vi "Interface Benchmark.vi"() -> (3 "one-way latency":u64 format="%d us")   [LabVIEW 2017]
uses:
  <vilib>/Platform/TimedLoop/XDataNode/timing_clust.ctl
  <vilib>/Platform/TimedLoop/XDataNode/nitl_modes.ctl
  <vilib>/Platform/TimedLoop/XDataNode/wakeup.ctl
  <vilib>/platform/TimedLoop/XDataNode/XDataNode.xnode
  Classes/Interfaces/Dispatcher/Dispatcher Interface.lvclass
  <vilib>/Platform/TimedLoop/XDataNode/XDNodeRunTimeDep.lvlib
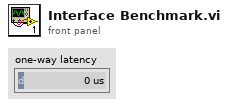
[diagram p1: front panel]
types:
  T1 = typedef "XDNodeRunTimeDep.lvlib/timing_clust.ctl" = cluster{"Expected End [f-1]":u64, "Actual End [f-1]":u64, "Finished Late? [f-1]":bool, "Expected End [i-1]":u64, "Actual End [i-1]":u64, "Finished Late? [i-1]":bool, "Expected Start [i]":u64, "Actual Start [i]":u64, "Expected Start [f]":u64, "Actual Start [f]":u64, "Source Name":string, "Structure Name":string, "Period":i64, "Deadline":i64, "Offset":i64, "Start":i64, "Priority":i32, "Timeout":i32, "Mode":T2, "Wakeup Reason":T3, "Error":errorcluster, "Source Type":string, "Secondary Source Type":string, "Global End Time":u64, "Global Start Time":u64, "Frame Duration":u64, "Iteration Duration":u64, "Assigned CPU":i32, "I/O Scan Engine Mode":u32}
  T2 = typedef "XDNodeRunTimeDep.lvlib/nitl_modes.ctl" = enum32{"No Change", "Process missed periods, maintain original phase", "Discard missed periods, maintain original phase", "Process missed periods, ignore original phase", "Discard missed periods, ignore original phase"}
  T3 = typedef "XDNodeRunTimeDep.lvlib/wakeup.ctl" = enum32{"Normal", "Aborted", "Asynchronous wakeup", "Timing source error", "Timed loop error", "Timeout"}
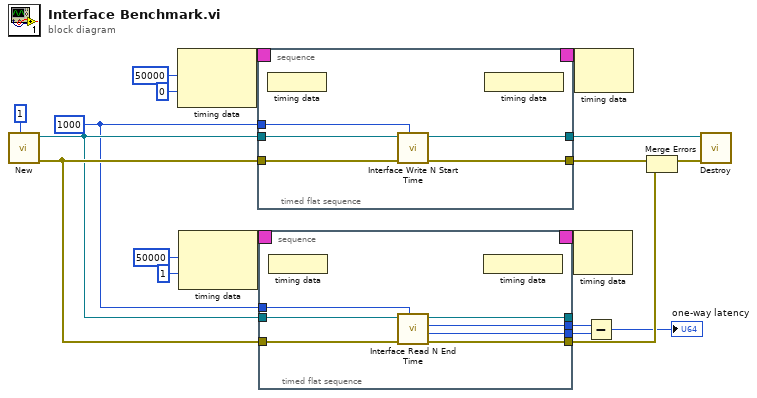
[diagram p0: block diagram]
diagram:
  w1 = 1000 ("count (1)")
  n1 = call "New.vi"("fifo depths (10)"=u32 1) -> ("error out"=w9:errorcluster, "Dispatcher Interface"=w8:refnum<class "Dispatcher Interface.lvclass">)  [unwired: 9 in]
  n2 = node-c288(50000 ("Priority"), 0 ("Processor")) -> (w15:T1)
  n3 = node-c288(50000 ("Priority"), 1 ("Processor")) -> (w12:T1)
  n4 = timed-sequence {
    timing: w15 -> [_]
    timing-out: [_] -> w14
    tunnel: [w24] -> w18
    tunnel: w9 -> [w23]
    tunnel: [w22] -> w17
    tunnel: w8 -> [w21]
    tunnel: w1 -> [w20]
    n5 = timed-flat-sequence {
      tunnel: [w29] -> w24
      tunnel: w23 -> [w28]
      tunnel: [w27] -> w22
      tunnel: w21 -> [w26]
      tunnel: w20 -> [w25]
      n6 = node-c288() -> ()  [unwired: 1 in]
      n7 = call "Interface Write N Start Time.vi"("count (1)"=w25, "error in (no error)"=w28, "Dispatcher Interface in"=w26) -> ("error out"=w27:errorcluster, "Dispatcher Interface out"=w29:refnum<class "Dispatcher Interface.lvclass">)  [unwired: 7 in]
      n8 = node-c288() -> ()  [unwired: 1 out]
    }
  }
  n9 = timed-sequence {
    timing: w12 -> [_]
    timing-out: [_] -> w11
    tunnel: [w38] -> _
    tunnel: w9 -> [w34]
    tunnel: [w37] -> w10
    tunnel: w8 -> [w33]
    tunnel: [w36] -> w6
    tunnel: [w35] -> w7
    tunnel: w1 -> [w32]
    n10 = timed-flat-sequence {
      tunnel: [w44] -> w38
      tunnel: [w45] -> w37
      tunnel: [w39] -> w36
      tunnel: [w43] -> w35
      tunnel: w34 -> [w42]
      tunnel: w33 -> [w41]
      tunnel: w32 -> [w40]
      n11 = node-c288() -> ()  [unwired: 1 in]
      n12 = call "Interface Read N End Time.vi"("count (1)"=w40, "error in (no error)"=w42, "Dispatcher Interface in"=w41) -> ("error out"=w45:errorcluster, "arg1"=w39:u64, "us count"=w43:u32, "Dispatcher Interface out"=w44:refnum<class "Dispatcher Interface.lvclass">)  [unwired: 5 in]
      n13 = node-c288() -> ()  [unwired: 1 out]
    }
  }
  n14 = node-c288(w11) -> ()  [unwired: 1 out]
  n15 = node-c288(w14) -> ()  [unwired: 1 out]
  n16 = Subtract(x=w7, y=w6) -> (x-y=→"one-way latency":u64)
  n17 = Merge Errors(w17, w10) -> (w16:errorcluster)
  n18 = call "Destroy.vi"("error in (no error)"=w16, "Dispatcher Interface in"=w18) -> ()  [unwired: 9 in, 1 out]
